vi "RIO Check.vi"(8 "error in":errorcluster, 11 "Requires RIO":bool) -> (0 "error out":errorcluster, 3 "RIO needed but not installed":bool)   [LabVIEW 2013]
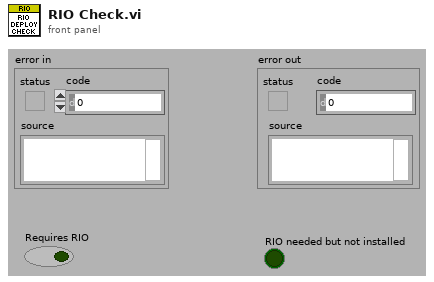
[diagram p1: front panel]
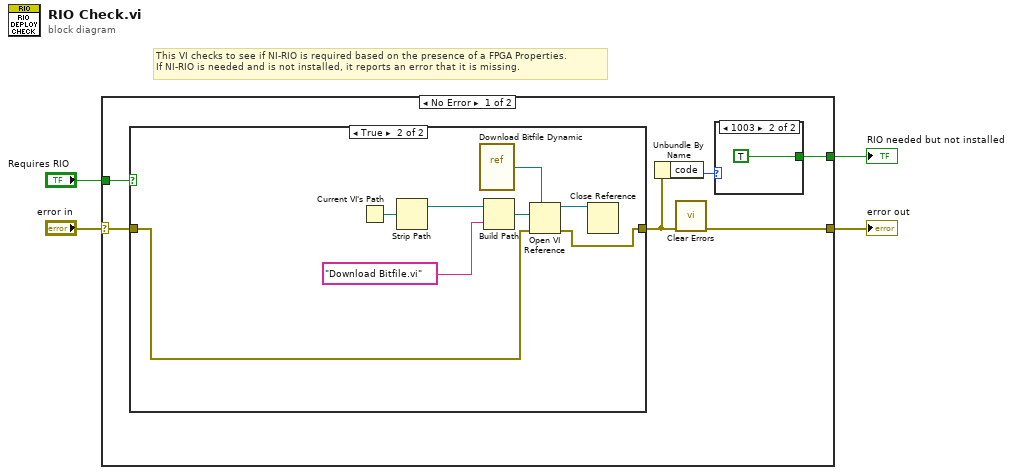
[diagram p0: block diagram]
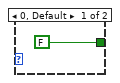
[diagram p2: hidden frame]
diagram:
  # "This VI checks to see if NI-RIO is required based on the presence of a FPGA Properties.\nIf NI-RIO is needed and is not installed, it reports an error that it is missing."
  n1 = case shown="No Error" "error in" {
    selector: "error in" -> [w6 w22]
    tunnel: "Requires RIO" -> [w10 _]
    tunnel: [w9 _] -> w3
    tunnel: [w5 w22] -> w2
    frame No Error {
      n2 = case shown="True" w10 {
        tunnel: w6 -> [w13 w15]
        tunnel: [w13 w17] -> w7
        frame False {
        }
        frame True {
          n3 = Current VI's Path() -> (path=w14:path)
          n4 = Strip Path(path=w14) -> (stripped path=w20:path)  [unwired: 1 out]
          n5 = vi-ref "Download Bitfile Dynamic.vi"() -> (w18:refnum<vi>)
          n6 = Build Path(base path=w20, name or relative path="Download Bitfile.vi") -> (appended path=w19:path)
          n7 = Open VI Reference(type specifier VI Refnum (for type only)=w18, vi path=w19, error in (no error)=w15) -> (vi reference=w16:refnum<vi>, error out=w17:errorcluster)  [unwired: 3 in]
          n8 = Close Reference(reference=w16) -> ()  [unwired: 1 in, 1 out]
        }
      }
      n9 = Unbundle By Name(w7) -> ("code"=w8:i32)
      n10 = call <vilib>:"Clear Errors.vi"("error in (no error)"=w7) -> ("error out"=w5:errorcluster)  [unwired: 6 in]
      n11 = case shown="1003" w8 {
        tunnel: [FALSE TRUE] -> w9
        frame 0, Default {
        }
        frame 1003 {
        }
      }
    }
    frame Error {
    }
  }
  "error out" <- w2
  "RIO needed but not installed" <- w3
